vi "Populate All Fields.vi"(8 "error in (no error)":errorcluster, 11 "Panel Form Controller in":refnum<class "Panel Form Controller.lvclass">) -> (0 "error out":errorcluster, 3 "Panel Form Controller out":refnum<class "Panel Form Controller.lvclass">)   [LabVIEW 2020, in "Panel Form Controller.lvlib" / "Panel Form Controller.lvclass"]
uses:
  Panel Form Controller.lvclass
  Panel Form Controller.lvclass/Panel Form Controller.ctl
  Database OOP/Table Libraries/Basic Form/Basic Form.lvclass
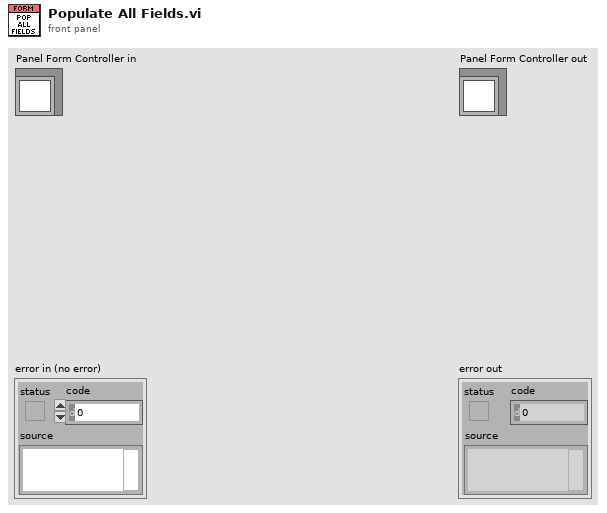
[diagram p1: front panel]
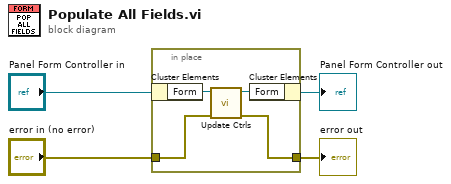
[diagram p0: block diagram]
diagram:
  n1 = in-place {
    in-place-border: "error in (no error)" -> [w6]
    in-place-border: [w5] -> w3
    n2 = in-place-cluster #1("Panel Form Controller in") -> ("Form"=w8:refnum<class "Basic Form.lvclass">)
    n3 = call "Update Ctrls.vi"("error in (no error)"=w6, "Basic Form in"=w8) -> ("error out"=w5:errorcluster, "Basic Form out"=w7:refnum<class "Basic Form.lvclass">)  [unwired: 8 in]
    n4 = in-place-cluster #1("Form"=w7) -> (→"Panel Form Controller out":refnum<class "Panel Form Controller.lvclass">)
  }
  "error out" <- w3
